vi "AlliGator Get Updated Phasor Ratio References.vi"(8 "error in (no error)":errorcluster) -> (0 "error out":errorcluster, 2 "Phasor Ratio Reference 2":T1, 3 "Phasor Ratio Reference 1":T1)   [LabVIEW 2021, in "AlliGator Phasor Ratio.lvlib"]
doc: "Updates references when the harmonic is changed."
uses:
  AlliGator Phasor Ratio.lvlib
  Phasor/Phasor (g, s).ctl
  Globals, Variables, Constants/AlliGator Variables List.ctl
  8b221e39-8fdf-4985-974c-e4e1025b3f2e.vi
  85322371-a0a8-493c-9dec-5fc54b1c0810.vi
  8b221e39-8fdf-4985-974c-e4e1025b3f2e.vi/8a80743f-1319-44c8-96b0-3ef8fc688731.vi
  8b221e39-8fdf-4985-974c-e4e1025b3f2e.vi/931f4f8f-d8c6-4056-833f-5c8fe97b24b9.vi
  85322371-a0a8-493c-9dec-5fc54b1c0810.vi/8a80743f-1319-44c8-96b0-3ef8fc688731.vi
  85322371-a0a8-493c-9dec-5fc54b1c0810.vi/931f4f8f-d8c6-4056-833f-5c8fe97b24b9.vi
  <vilib>/Utility/error.llb/Error Cluster From Error Code.vi
  <vilib>/ErrorRing/Error Ring.xnode
  Phasor/Phasor.lvlib
  Globals, Variables, Constants/AlliGator Globals, Variables & Constants.lvlib
  Settings/AlliGator Settings.lvlib
panel:
  # "see the AlliGator License on the block diagram (Ctrl+E or Window:Show Block Diagram)"
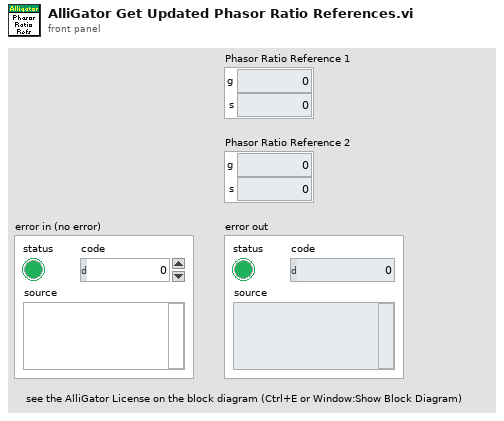
[diagram p1: front panel]
types:
  T1 = typedef "Phasor.lvlib/Phasor (g, s).ctl" = cluster{"g":dbl, "s":dbl}
  T2 = typedef "AlliGator Globals, Variables & Constants.lvlib/AlliGator Variables List.ctl" = enum16{"---- GUI ----", "GUI:Initialization Status", "GUI:State Indicators Refnum", "GUI:Original AlliGator Menu Items", "GUI:Current Action Loop State", "GUI:Script in progress", "GUI:Playback", "GUI:Loop Playback", "GUI:Search ROI Used", "GUI:Search ROI", "Decay Graph Max Legend Size", "Intensity Graph Max Legend Size", "Decay Statistics Graph Max Legend Size", "Phasor Graph Max Legend Size", "Phasor Ratio Graph Max Legend Size", "Lifetime Graph Max Legend Size", "---- Files ----", "Files:Export Dataset Frames as Individual Files", "Files:Show Batch Export Help Balloons", "Files:Frames in Dataset", "Files:ptu File Frame Start Indices", "Files:Current Frame in Dataset", "Files:Current Frame Timestamp", "Files:Dataset Loaded", "Files:Dataset Metadata", "Files:Dataset Channel", "Files:Dataset Data Description", "Files:Background Dataset Metadata", "Files:Background Dataset Channel", "Files:Background Dataset Data Description", "Files:Background File Subtraction", "Files:Background File Path", "Files:Background File Pile-up Correction", "Files:Background File Pixel Well Capacity", "Files:Background File Scaling Factor", "Files:Current Dataset Load Settings", "Files:Dataset Path", "Files:ICCD-specific Information", "Files:Macrotime Gate Separation", "------ Python Plugins ------", "Python Plugins:Information", "Python Plugins:Python Session", "Python Plugins:Valid Python Session?", "---- Source Image ----", "Source Image:ROIs", "Source Image:Current ROI", "Source Image:ROI Event Refnum", "X_Source Image Display Range", "X_Source Image Palette Information", "X_Type of Displayed Image", "X_Time Gate Slider", "Source Image:Palette List", "Source Image:Scale", "Source Image:ROI Overlay Color", "Source Image:Overlay to Erase", "Source Image:Is Displayed Image Accumulated", "Source Image:White Light Image Modified", "Source Image:Mask Image Modified", "---- Image Profile Window ----", "Image Profile:Window Event Refnum", "Image Profile:IntensityType", "Image Profile:Intensity Average Type", "Image Profile:Intensity-weighted SDV", "Image Profile:Box Profile Type", "Image Profile:Window Open", "Image Profile:Plotted Fit Parameter", "------ Phasor Graph -------", "Phasor Graph:Show Line", "---- Phasor Plot ---", "Phasor Plot:Parameters Changed", "Phasor Plot:FLI Dataset Modified since last Calculation", "Phasor Harmonics Data", "Selected Phasor Harmonics", "Phasor Harmonic Manager Event Refnum", "Phasor Plot:ROIs", "Phasor Plot:Current ROI", "Phasor Plot:ROI Event Refnum", "Phasor Plot:Image Reference Points", "Phasor Plot:Computed", "Phasor Plot:Palette Information", "Phasor Plot:Palette List", "Phasor Plot:Phasor Ratio Palette Information", "Phasor Plot:Phasor Ratio Palette List", "Phasor Plot:Image Scale", "Phasor Plot:Image Overlay to Erase", "Phasor Plot:Image Elements to Update", "Phasor Plot:Current Calculation Parameters", "Phasor Plot:Current Calibration Options", "Phasor Plot:Reset Cumulated Phasor Plot", "Phasor Plot:Reference 1", "Phasor Plot:Lifetime Reference 1", "Phasor Plot:Reference 1 Frequency", "Phasor Plot:Reference 2", "Phasor Plot:Lifetime Reference 2", "Phasor Plot:Reference 2 Frequency", "---- Decay Analysis ----", "Number of Selected Decays to Fit", "LS Fit Results", "LAR Fit Results", "BS Fit Results", "Last Decay Max - Min", "Best Fit Parameters", "Best Fit Parameter Names", "Actual Size X", "Actual Size Y", "Binning X", "Binning Y", "Actual # Gates", "Dataset Number", "Gates to...", "Gates Skipped", "Gates to keep", "Gate Step", "Gate Separation", "Reversed Gates", "Pile-up Correction", "Pixel Well Capacity", "Background Subtracted", "Background Subtraction Method", "Background Definition Range", "Background File (deprecated)", "Number of Dataset Accumulated", "Array of Accumulated Dataset Paths", "Do Averaged Datasets", "Destination File Path", "Process Plot Target", "Use 1/D as Phasor Frequency", "---- Decay Fit Parameter Map -----", "Decay Fit Parameter Map:Palette Information", "Decay Fit Parameter Map:Palette List", "---- Parameter Map ----", "Parameter Map:Palette Information", "Parameter Map:Palette List", "------- Local Decay Window ---------", "Local Decay Graph Window:Event Refnum", "Local Decay Graph Window:Use normalized IRF for convolution", "----- Miscellaneous ----", "Misc:Skippable Dialog Windows Status"}
  T3 = typedef "Phasor.lvlib/Phasor (m, phi).ctl" = cluster{"m":dbl, "phi":dbl}
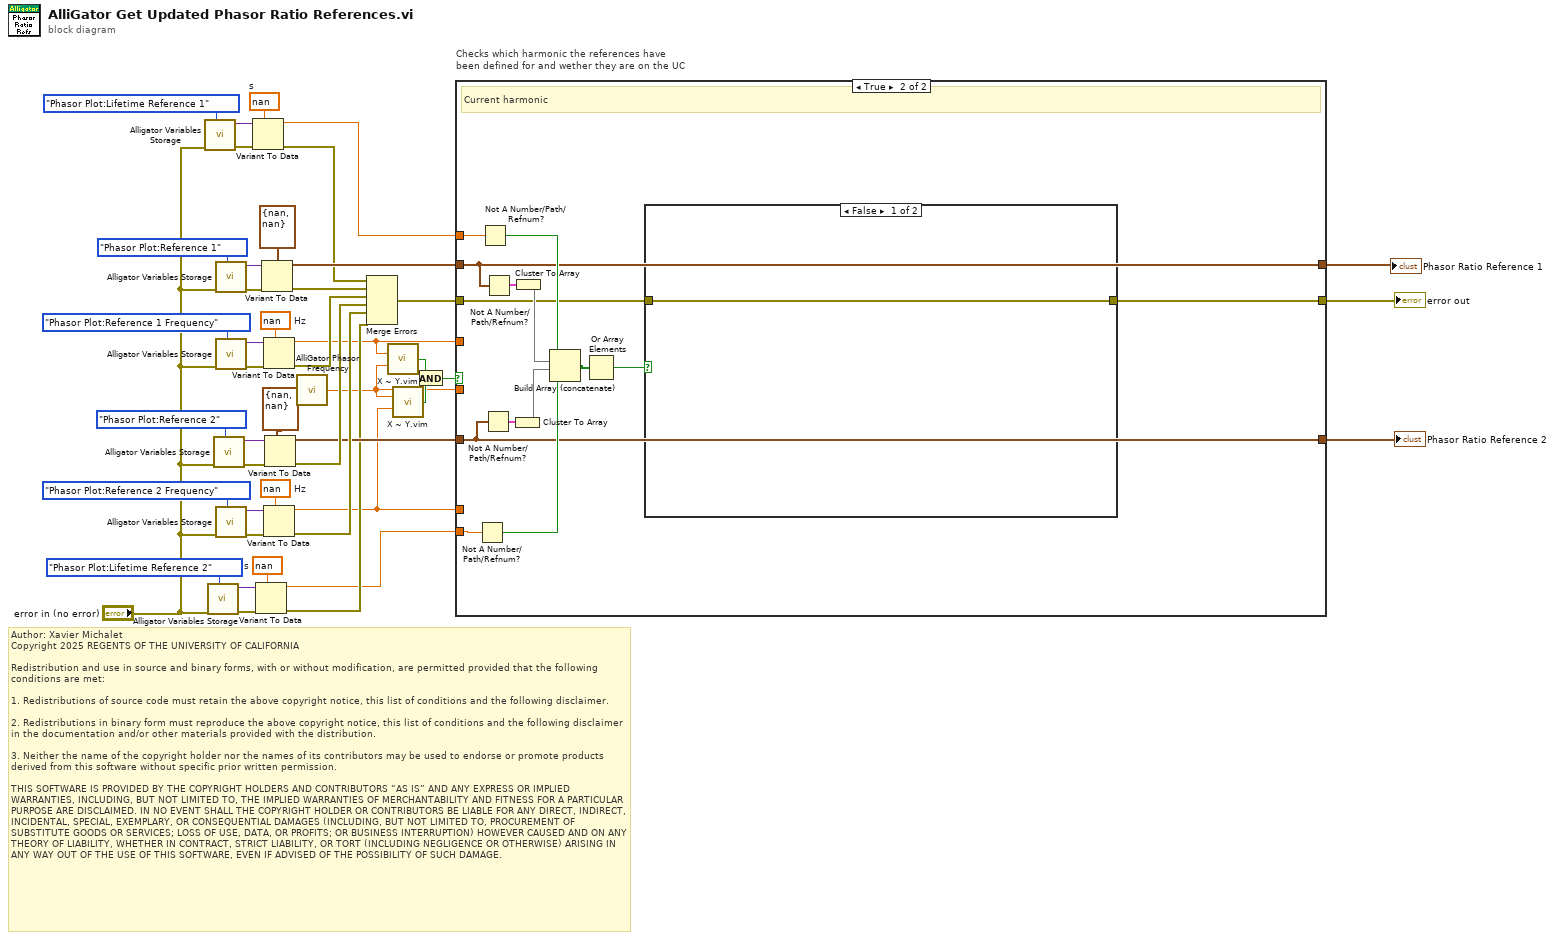
[diagram p0: block diagram]
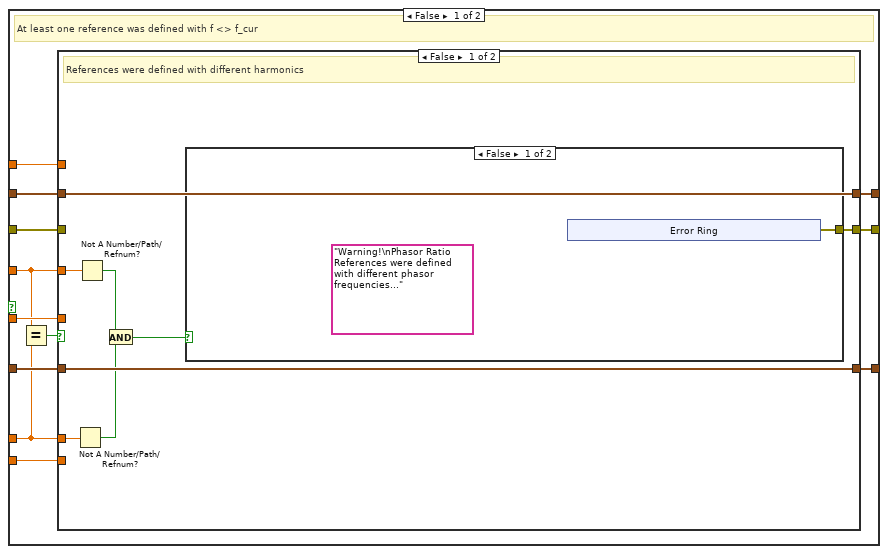
[diagram p2: hidden frame]
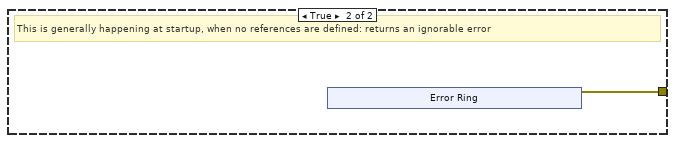
[diagram p3: hidden frame]
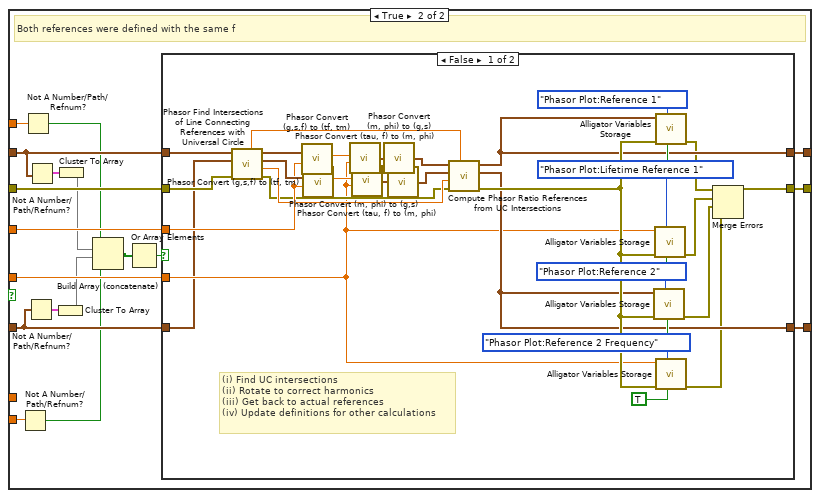
[diagram p4: hidden frame]
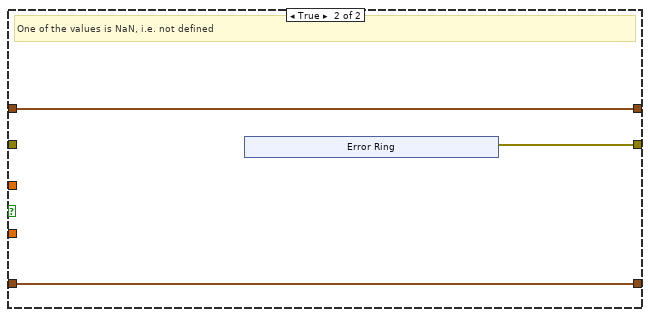
[diagram p5: hidden frame]
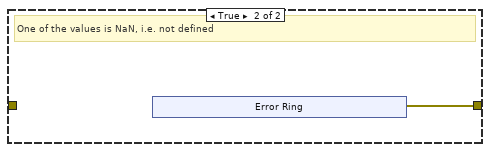
[diagram p6: hidden frame]
diagram:
  w9 = dbl[unit] nan  # s
  w16 = dbl[unit] nan  # s
  w32 = dbl[unit] nan  # Hz
  w33 = dbl[unit] nan  # Hz
  # "Author: Xavier Michalet\nCopyright 2025 REGENTS OF THE UNIVERSITY OF CALIFORNIA\n\nRedistribution and use in source and binary forms, with or without modification, are permitted provided that the following conditions are met:\n\n1. Redistributions of source code must retain the above copyright notice, this list of conditions and the following disclaimer.\n\n2. Redistributions in binary form must reproduce the above copyright notice, this list of conditions and the following disclaimer in the documentation and/or other materials provided with the distribution.\n\n3. Neither the name of the copyright holder nor the names of its contributors may be used to endorse or promote products derived from this software without specific prior written permission.\n\nTHIS SOFTWARE IS PROVIDED BY THE COPYRIGHT HOLDERS AND CONTRIBUTORS “AS IS” AND ANY EXPRESS OR IMPLIED WARRANTIES, INCLUDING, BUT NOT LIMITED TO, THE IMPLIED WARRANTIES OF MERCHANTABILITY AND FITNESS FOR A PARTICULAR PURPOSE ARE DISCLAIMED. IN NO EVENT SHALL THE COPYRIGHT HOLDER OR CONTRIBUTORS BE LIABLE FOR ANY DIRECT, INDIRECT, INCIDENTAL, SPECIAL, EXEMPLARY, OR CONSEQUENTIAL DAMAGES (INCLUDING, BUT NOT LIMITED TO, PROCUREMENT OF SUBSTITUTE GOODS OR SERVICES; LOSS OF USE, DATA, OR PROFITS; OR BUSINESS INTERRUPTION) HOWEVER CAUSED AND ON ANY THEORY OF LIABILITY, WHETHER IN CONTRACT, STRICT LIABILITY, OR TORT (INCLUDING NEGLIGENCE OR OTHERWISE) ARISING IN ANY WAY OUT OF THE USE OF THIS SOFTWARE, EVEN IF ADVISED OF THE POSSIBILITY OF SUCH DAMAGE."
  n1 = call "Alligator Variables Storage.vi"("AlliGator Variable"=AlliGator_Variables_List."Phasor Plot:Lifetime Reference 1" ("Alligator Variable"), "Error In"="error in (no error)") -> ("Error Out"=w14:errorcluster, "Data out"=w15:variant)  [unwired: 7 in, 1 out]
  n2 = call "Alligator Variables Storage.vi"("AlliGator Variable"=AlliGator_Variables_List."Phasor Plot:Lifetime Reference 2" ("Alligator Variable"), "Error In"="error in (no error)") -> ("Error Out"=w7:errorcluster, "Data out"=w10:variant)  [unwired: 7 in, 1 out]
  n3 = call "Alligator Variables Storage.vi"("AlliGator Variable"=AlliGator_Variables_List."Phasor Plot:Reference 2" ("Alligator Variable"), "Error In"="error in (no error)") -> ("Error Out"=w39:errorcluster, "Data out"=w38:variant)  [unwired: 7 in, 1 out]
  n4 = call "Alligator Variables Storage.vi"("AlliGator Variable"=AlliGator_Variables_List."Phasor Plot:Reference 1" ("Alligator Variable"), "Error In"="error in (no error)") -> ("Error Out"=w42:errorcluster, "Data out"=w43:variant)  [unwired: 7 in, 1 out]
  n5 = call "Alligator Variables Storage.vi"("AlliGator Variable"=AlliGator_Variables_List."Phasor Plot:Reference 1 Frequency" ("Alligator Variable"), "Error In"="error in (no error)") -> ("Error Out"=w35:errorcluster, "Data out"=w34:variant)  [unwired: 7 in, 1 out]
  n6 = call "Alligator Variables Storage.vi"("AlliGator Variable"=AlliGator_Variables_List."Phasor Plot:Reference 2 Frequency" ("Alligator Variable"), "Error In"="error in (no error)") -> ("Error Out"=w30:errorcluster, "Data out"=w31:variant)  [unwired: 7 in, 1 out]
  n7 = Variant To Data(error in=w14, type=w16, Variant=w15) -> (data=w5:dbl[unit], error out=w12:errorcluster)
  n8 = Variant To Data(error in=w7, type=w9, Variant=w10) -> (data=w4:dbl[unit], error out=w6:errorcluster)
  n9 = Variant To Data(error in=w42, type=T1 {"g"=nan, "s"=nan} ("Phasor Ratio Reference 1"), Variant=w43) -> (data=w22:T1, error out=w45:errorcluster)
  n10 = Variant To Data(error in=w35, type=w33, Variant=w34) -> (data=w3:dbl[unit], error out=w28:errorcluster)
  n11 = Variant To Data(error in=w30, type=w32, Variant=w31) -> (data=w1:dbl[unit], error out=w26:errorcluster)
  n12 = Variant To Data(error in=w39, type=T1 {"g"=nan, "s"=nan} ("Phasor Ratio Reference 1"), Variant=w38) -> (data=w20:T1, error out=w27:errorcluster)
  n13 = call "AlliGator Phasor Frequency.vi"() -> ("Phasor Frequency"=w2:dbl[unit])
  n14 = Merge Errors(w12, w45, w28, w27, w26, w6) -> (w18:errorcluster)
  n15 = call "X ~ Y.vim"("X"=w3, "Y"=w2) -> ("X ~= Y?"=w25:bool)  [unwired: 13 in]
  n16 = call "X ~ Y.vim"("X"=w2, "Y"=w1) -> ("X ~= Y?"=w24:bool)  [unwired: 13 in]
  n17 = And(x=w25, y=w24) -> (x .and. y?=w23:bool)
  n18 = case "Checks which harmonic the references have been defined for and wether they are on the UC" shown="True" w23 {
    tunnel: w22 -> [w56 w135]
    tunnel: [w49 w135] -> w21
    tunnel: w20 -> [w55 w134]
    tunnel: [w47 w134] -> w19
    tunnel: w18 -> [w54 w130]
    tunnel: [w48 w131] -> w17
    tunnel: w1 -> [w46 _]
    tunnel: w3 -> [w50 _]
    tunnel: w5 -> [w53 w136]
    tunnel: w4 -> [w52 w133]
    tunnel: w2 -> [w51 _]
    frame False {
      # "At least one reference was defined with f <> f_cur"
      n19 = Equal?(x=w50, y=w46) -> (x = y?=w57:bool)
      n20 = case shown="False" w57 {
        tunnel: w56 -> [w65 w85]
        tunnel: w55 -> [w64 w84]
        tunnel: w54 -> [_ w93]
        tunnel: w53 -> [_ w87]
        tunnel: w52 -> [_ w86]
        tunnel: w51 -> [_ w89]
        tunnel: w50 -> [w62 w92]
        tunnel: [w65 w91] -> w49
        tunnel: [w63 w88] -> w48
        tunnel: [w64 w90] -> w47
        tunnel: w46 -> [w61 _]
        frame False {
          # "References were defined with different harmonics"
          n21 = Not A Number/Path/Refnum?(number/path/refnum=w61) -> (NaN/Path/Refnum?=w59:bool)
          n22 = Not A Number/Path/Refnum?(number/path/refnum=w62) -> (NaN/Path/Refnum?=w60:bool)
          n23 = And(x=w60, y=w59) -> (x .and. y?=w58:bool)
          n24 = case shown="False" w58 {
            tunnel: [w66 w71] -> w63
            frame False {
              (unwired) "Warning!\nPhasor Ratio References were defined with different phasor frequencies..." ("message")
              n25 = xnode "Error Ring"() -> ("error out"=w66:errorcluster)
            }
            frame True {
              # "This is generally happening at startup, when no references are defined: returns an ignorable error"
              n26 = xnode "Error Ring"() -> ("error out"=w71:errorcluster)
            }
          }
        }
        frame True {
          # "Both references were defined with the same f"
          n27 = Not A Number/Path/Refnum?(number/path/refnum=w86) -> (NaN/Path/Refnum?=w78:bool)
          n28 = Not A Number/Path/Refnum?(number/path/refnum=w87) -> (NaN/Path/Refnum?=w81:bool)
          n29 = Not A Number/Path/Refnum?(number/path/refnum=w84) -> (NaN/Path/Refnum?=w82:cluster{"g":bool, "s":bool})
          n30 = Not A Number/Path/Refnum?(number/path/refnum=w85) -> (NaN/Path/Refnum?=w83:cluster{"g":bool, "s":bool})
          n31 = Cluster To Array(cluster=w82) -> (array=w79:bool[])
          n32 = Cluster To Array(cluster=w83) -> (array=w80:bool[])
          n33 = Build Array (concatenate)(w81, w80, w79, w78) -> (w77:bool[])
          n34 = Or Array Elements(Boolean array=w77) -> (logical OR=w76:bool)
          n35 = case shown="False" w76 {
            tunnel: w93 -> [w122 _]
            tunnel: w92 -> [w118 _]
            tunnel: [w103 w125] -> w91
            tunnel: [w102 w124] -> w90
            tunnel: w89 -> [w101 _]
            tunnel: [w96 w123] -> w88
            tunnel: w85 -> [w95 w125]
            tunnel: w84 -> [w94 w124]
            frame False {
              w104 = TRUE ("Get(F)/Set")
              # "(i) Find UC intersections\n(ii) Rotate to correct harmonics\n(iii) Get back to actual references\n(iv) Update definitions for other calculations"
              n36 = call "Phasor Find Intersections of Line Connecting References with Universal Circle.vi"("Error In"=w122, "Phasor 2"=w94, "Phasor 1"=w95) -> ("Error Out"=w115:errorcluster, "mu-"=w116:dbl, "Intersection 2"=w119:cluster{"x":dbl, "y":dbl}, "Intersection 1"=w121:cluster{"x":dbl, "y":dbl}, "mu+"=w110:dbl)  [unwired: 4 in]
              n37 = call "Phasor Convert (g,s,f) to (tf, tm).vi"("Phasor Harmonic Frequency"=w118, "Phasor (g, s)"=w121) -> ("Phase Lifetime"=w120:dbl[unit])  [unwired: 7 in, 2 out]
              n38 = call "Phasor Convert (g,s,f) to (tf, tm).vi"("Phasor Harmonic Frequency"=w118, "Phasor (g, s)"=w119) -> ("Phase Lifetime"=w117:dbl[unit])  [unwired: 7 in, 2 out]
              n39 = call "Phasor Convert (tau, f) to (m, phi).vi"("Lifetime"=w120, "Phasor Frequency"=w101) -> ("Phasor (m, phi)"=w114:T3)  [unwired: 5 in]
              n40 = call "Phasor Convert (tau, f) to (m, phi).vi"("Lifetime"=w117, "Phasor Frequency"=w101) -> ("Phasor (m, phi)"=w112:T3)  [unwired: 5 in]
              n41 = call "Phasor Convert (m, phi) to (g,s).vi"("Phasor (m, phi)"=w114) -> ("Phasor (g, s)"=w113:T1)  [unwired: 8 in]
              n42 = call "Phasor Convert (m, phi) to (g,s).vi"("Phasor (m, phi)"=w112) -> ("Phasor (g, s)"=w111:T1)  [unwired: 8 in]
              n43 = call "Compute Phasor Ratio References from UC Intersections.vi"("mu+"=w110, "error in (no error)"=w115, "mu-"=w116, "Phasor 1 (g, s)"=w111, "Phasor 2 (g, s)"=w113) -> ("error out"=w105:errorcluster, "Reference Phasor 2 (g, s)"=w102:T1, "Reference Phasor 1 (g, s)"=w103:T1)  [unwired: 4 in]
              n44 = call "Alligator Variables Storage.vi"("Get(F)/Set"=w104, "AlliGator Variable"=AlliGator_Variables_List."Phasor Plot:Reference 2" ("Alligator Variable"), "Error In"=w105, "Data in"=w102) -> ("Error Out"=w99:errorcluster)  [unwired: 5 in, 2 out]
              n45 = call "Alligator Variables Storage.vi"("Get(F)/Set"=w104, "AlliGator Variable"=AlliGator_Variables_List."Phasor Plot:Lifetime Reference 1" ("Alligator Variable"), "Error In"=w105, "Data in"=w101) -> ("Error Out"=w98:errorcluster)  [unwired: 5 in, 2 out]
              n46 = call "Alligator Variables Storage.vi"("Get(F)/Set"=w104, "AlliGator Variable"=AlliGator_Variables_List."Phasor Plot:Reference 1" ("Alligator Variable"), "Error In"=w105, "Data in"=w103) -> ("Error Out"=w97:errorcluster)  [unwired: 5 in, 2 out]
              n47 = call "Alligator Variables Storage.vi"("Get(F)/Set"=w104, "AlliGator Variable"=AlliGator_Variables_List."Phasor Plot:Reference 2 Frequency" ("Alligator Variable"), "Error In"=w105, "Data in"=w101) -> ("Error Out"=w100:errorcluster)  [unwired: 5 in, 2 out]
              n48 = Merge Errors(w97, w98, w99, w100) -> (w96:errorcluster)
            }
            frame True {
              # "One of the values is NaN, i.e. not defined"
              n49 = xnode "Error Ring"() -> ("error out"=w123:errorcluster)
            }
          }
        }
      }
    }
    frame True {
      # "Current harmonic"
      n50 = Not A Number/Path/Refnum?(number/path/refnum=w133) -> (NaN/Path/Refnum?=w138:bool)
      n51 = Not A Number/Path/Refnum?(number/path/refnum=w136) -> (NaN/Path/Refnum?=w141:bool)
      n52 = Not A Number/Path/Refnum?(number/path/refnum=w134) -> (NaN/Path/Refnum?=w142:cluster{"g":bool, "s":bool})
      n53 = Not A Number/Path/Refnum?(number/path/refnum=w135) -> (NaN/Path/Refnum?=w143:cluster{"g":bool, "s":bool})
      n54 = Cluster To Array(cluster=w142) -> (array=w139:bool[])
      n55 = Cluster To Array(cluster=w143) -> (array=w140:bool[])
      n56 = Build Array (concatenate)(w141, w140, w139, w138) -> (w137:bool[])
      n57 = Or Array Elements(Boolean array=w137) -> (logical OR=w132:bool)
      n58 = case shown="False" w132 {
        tunnel: [w144 w145] -> w131
        tunnel: w130 -> [w144 _]
        frame False {
        }
        frame True {
          # "One of the values is NaN, i.e. not defined"
          n59 = xnode "Error Ring"() -> ("error out"=w145:errorcluster)
        }
      }
    }
  }
  "Phasor Ratio Reference 1" <- w21
  "Phasor Ratio Reference 2" <- w19
  "error out" <- w17
